vi "DBGetCopyFileList.vi"(8 "error in (no error)":errorcluster, 9 "message value":variant, 11 "ProcessState in":T1) -> (0 "error out":errorcluster, 1 "FilePaths":path[](array[path]), 3 "ProcessState out":T1)   [LabVIEW 2015, in "FileHandler.lvlib"]
uses:
  FileHandler.lvlib
  controls/ProcessState.ctl
  <vilib>/drjdpowell/SQLite Library/SQL Connection/Connection.lvclass
  <vilib>/drjdpowell/SQLite Library/SQL Statement/SQL Statement.lvclass/SQL Statement.ctl
  <vilib>/drjdpowell/SQLite Library/SQL Statement/Error Message.vi
  <vilib>/drjdpowell/SQLite Library/SQL Statement/Column Path.vi
  <vilib>/drjdpowell/SQLite Library/SQL Statement/SQL Statement.lvclass
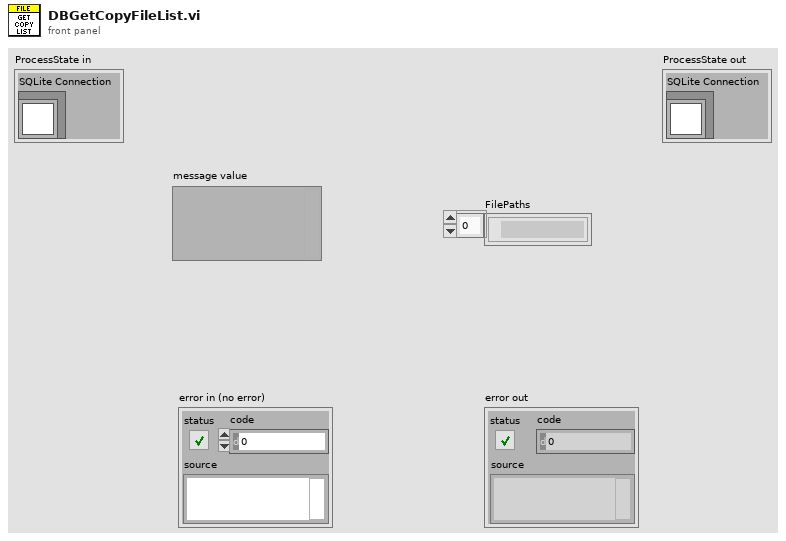
[diagram p1: front panel]
types:
  T1 = typedef "FileHandler.lvlib/ProcessState.ctl" = cluster{"SQLite Connection":refnum<class "Connection.lvclass">}
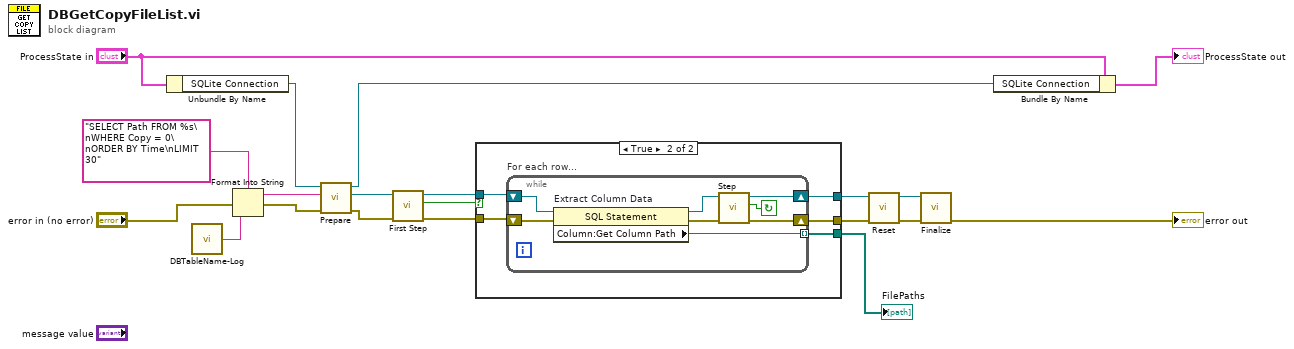
[diagram p0: block diagram]
diagram:
  n1 = Unbundle By Name("ProcessState in") -> ("SQLite Connection"=w15:refnum<class "Connection.lvclass">)
  n2 = call "DBTableName-Log.vi"() -> ("DB Table Name"=w17:string)  [unwired: 5 in]
  n3 = Format Into String(format string="SELECT Path FROM %s\nWHERE Copy = 0\nORDER BY Time\nLIMIT 30", error in="error in (no error)", w17) -> (resulting string=w16:string, error out=w4:errorcluster)  [unwired: 1 in]
  n4 = call <vilib>:"Prepare.vi"("error in (no error)"=w4, "SQL"=w16, "SQLite Connection in"=w15) -> ("error out"=w3:errorcluster, "SQL Statement out"=w14:refnum<class "SQL Statement.lvclass">, "SQLite Connection out"=w6:refnum<class "Connection.lvclass">)  [unwired: 4 in, 2 out]
  n5 = call <vilib>:"First Step.vi"("error in (no error)"=w3, "SQL Statement in"=w14) -> ("error out"=w8:errorcluster, "Row returned"=w7:bool, "SQL Statement out"=w9:refnum<class "SQL Statement.lvclass">)  [unwired: 7 in]
  n6 = case shown="True" w7 {
    tunnel: w9 -> [w21 w27]
    tunnel: w8 -> [w22 w26]
    tunnel: [w22 w25] -> w10
    tunnel: [w21 w24] -> w11
    tunnel: [_ w23] -> w1
    frame False {
    }
    frame True {
      n7 = while "For each row..." {
        shift-right: [w34] -> w24
        shift-left: w27 -> [w31]
        shift-right: [w32] -> w25
        shift-left: w26 -> [w30]
        tunnel: [w28] -> w23 mode=indexing
        stop <- w29 continue-if-true
        n8 = property on="Extract Column Data" class="SQL Statement"(reference=w31, error in=w30) -> (reference out=w35:refnum<class "SQL Statement.lvclass">, error out=w33:errorcluster, "Column:Get Column Path"=w28:path)
        n9 = call <vilib>:"Step.vi"("error in (no error)"=w33, "SQL Statement in"=w35) -> ("error out"=w32:errorcluster, "Row returned"=w29:bool, "SQL Statement out"=w34:refnum<class "SQL Statement.lvclass">)  [unwired: 7 in]
      }
    }
  }
  "FilePaths" <- w1
  n10 = call <vilib>:"Reset.vi"("error in (no error)"=w10, "SQL Statement in"=w11) -> ("error out"=w12:errorcluster, "SQL Statement out"=w13:refnum<class "SQL Statement.lvclass">)  [unwired: 8 in]
  n11 = call <vilib>:"Finalize.vi"("error in (no error)"=w12, "SQL Statement in"=w13) -> ("error out"=→"error out":errorcluster)  [unwired: 9 in]
  n12 = Bundle By Name(cluster="ProcessState in", "SQLite Connection"=w6) -> (→"ProcessState out":T1)
